vi "Configure Waveform Modulation (FM).vi"(6 "FM Frequency (1000 Hz)":dbl=1000.0, 8 "error in (no error)":errorcluster, 9 "FM Frequency Deviation (1000 Hz)":dbl=1000.0, 10 "Waveform Generator Number (1: Waveform Generator 1)":i32(ring)=1 items=["Waveform Generator 1"=1], 11 "VISA resource name":refnum<visa-resource-name>) -> (0 "error out":errorcluster, 3 "VISA resource name out":refnum<visa-resource-name>)   [LabVIEW 2015, in "Agilent 2000 3000 X-Series.lvlib"]
doc: "Configures the waveform modulation FM."
uses:
  Agilent 2000 3000 X-Series.lvlib
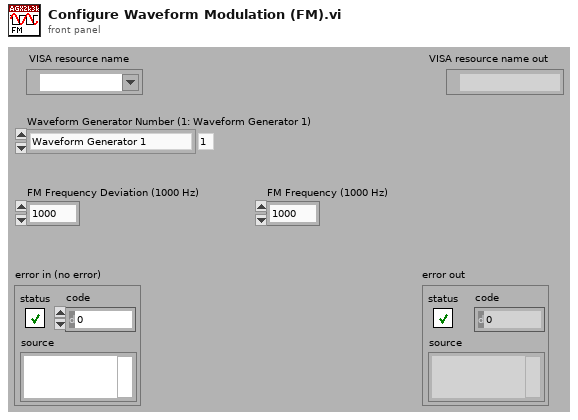
[diagram p1: front panel]
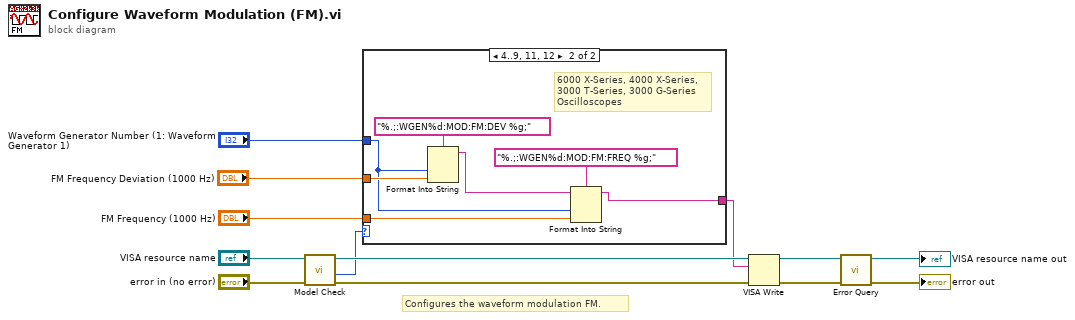
[diagram p0: block diagram]
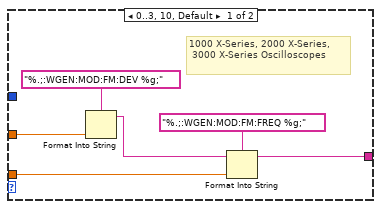
[diagram p2: hidden frame]
diagram:
  # "Configures the waveform modulation FM."
  n1 = call "Model Check.vi"("error in (no error)"="error in (no error)", "VISA resource name"="VISA resource name") -> ("error out"=w6:errorcluster, "Model"=w5:i32, "VISA resource name out"=w7:refnum<visa-resource-name>)  [unwired: 7 out]
  n2 = case shown="4..9, 11, 12" w5 {
    tunnel: "FM Frequency (1000 Hz)" -> [w15 w22]
    tunnel: "FM Frequency Deviation (1000 Hz)" -> [w16 w23]
    tunnel: "Waveform Generator Number (1: Waveform Generator 1)" -> [_ w20]
    tunnel: [w14 w21] -> w1
    frame 0..3, 10, Default {
      # "1000 X-Series, 2000 X-Series,\n 3000 X-Series Oscilloscopes"
      n3 = Format Into String(format string="%.;:WGEN:MOD:FM:DEV %g;", w16) -> (resulting string=w17:string)  [unwired: 2 in, 1 out]
      n4 = Format Into String(format string="%.;:WGEN:MOD:FM:FREQ %g;", initial string=w17, w15) -> (resulting string=w14:string)  [unwired: 1 in, 1 out]
    }
    frame 4..9, 11, 12 {
      # "6000 X-Series, 4000 X-Series, 3000 T-Series, 3000 G-Series Oscilloscopes"
      n5 = Format Into String(format string="%.;:WGEN%d:MOD:FM:DEV %g;", w20, w23) -> (resulting string=w24:string)  [unwired: 2 in, 1 out]
      n6 = Format Into String(format string="%.;:WGEN%d:MOD:FM:FREQ %g;", initial string=w24, w20, w22) -> (resulting string=w21:string)  [unwired: 1 in, 1 out]
    }
  }
  n7 = VISA Write(VISA resource name=w7, write buffer=w1, error in (no error)=w6) -> (VISA resource name out=w13:refnum<visa-resource-name>, error out=w12:errorcluster)  [unwired: 1 out]
  n8 = call "Error Query.vi"("error in (no error)"=w12, "VISA resource name"=w13) -> ("error out"=→"error out":errorcluster, "VISA resource name out"=→"VISA resource name out":refnum<visa-resource-name>)  [unwired: 6 in, 2 out]
